vi "JSON to LVObject - Error in Serializable Class - Returns Object Type.vi"() -> ()   [LabVIEW 2017, in "JSON Serializable Serializer Tests.lvlib"]
uses:
  JSON Serializable Serializer Tests.lvlib
  JSON Serializable Serializer/JSON Serializable Serializer.lvclass
  <vilib>/Utility/error.llb/Error Cluster From Error Code.vi
  <vilib>/addons/_JKI Toolkits/Caraya/classes/Assert/Assert Equal Value_Variant.vi
  <vilib>/ErrorRing/Error Ring.xnode
  <vilib>/addons/_JKI Toolkits/Caraya/classes/Test/Test.lvclass
  <vilib>/addons/_JKI Toolkits/Caraya/classes/Assert/Assert.lvclass
  Mock JSON Serializable/Mock JSON Serializable.lvclass
panel:
  out "error out":errorcluster
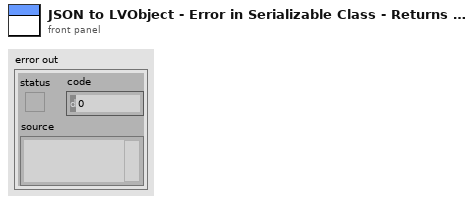
[diagram p1: front panel]
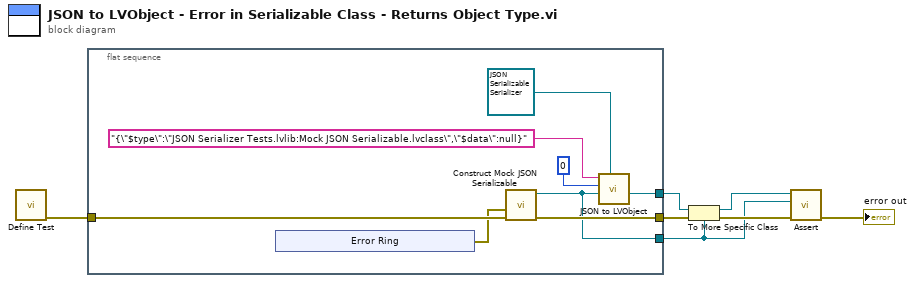
[diagram p0: block diagram]
diagram:
  n1 = call <vilib>:"Define Test.vi"() -> ("error out"=w7:errorcluster)  [unwired: 11 in]
  n2 = flat-sequence {
    tunnel: [w11] -> w5
    tunnel: w7 -> [w12]
    tunnel: [w9] -> w3
    tunnel: [w8] -> w1
    frame #0 {
      n3 = xnode "Error Ring"() -> ("error out"=w10:errorcluster)
      n4 = call "Construct Mock JSON Serializable.vi"("error in (no error)"=w12, "From/To JSON <error out> (no error)"=w10) -> ("error out"=w11:errorcluster, "Mock JSON Serializable"=w8:refnum<class "Mock JSON Serializable.lvclass">)  [unwired: 8 in]
      n5 = call-dynamic "JSON to LVObject.vi"("JSON Serializer in"=refnum<class "JSON Serializable Serializer.lvclass"> refnum ("JSON Serializer.lvclass"), "Object Type"=w8, "Offset"=0, "JSON"="{\"$type\":\"JSON Serializer Tests.lvlib:Mock JSON Serializable.lvclass\",\"$data\":null}") -> ("Object"=w9:refnum<class>)  [unwired: 6 in, 1 out]
    }
  }
  n6 = To More Specific Class(target class=w1, reference=w3, error in=w5) -> (specific class reference=w2:refnum<class "Mock JSON Serializable.lvclass">, error out=w4:errorcluster)
  n7 = call-poly <vilib>:"Assert.vi"("error in (no error)"=w4, "Y"=w1, "X"=w2) -> ("error out"=→"error out":errorcluster)  [unwired: 8 in]
